vi "Day11-1.vi"() -> ()   [LabVIEW 2021]
panel:
  out "Flashes":i32
  out "Array":i32[][](array[numeric])
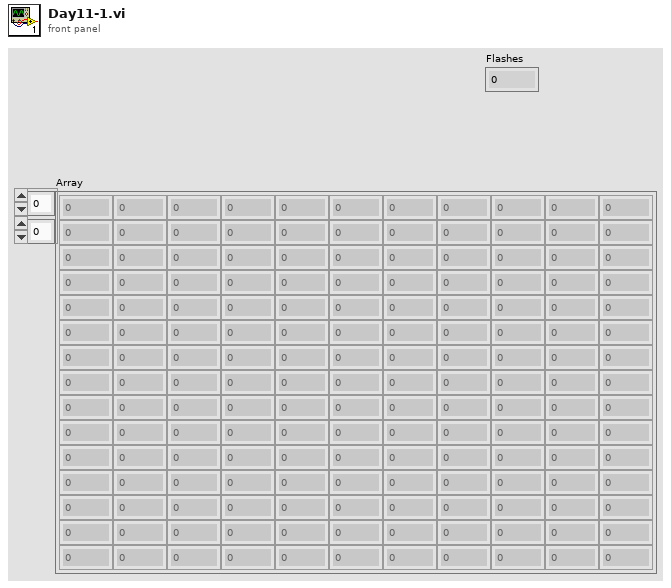
[diagram p1: front panel]
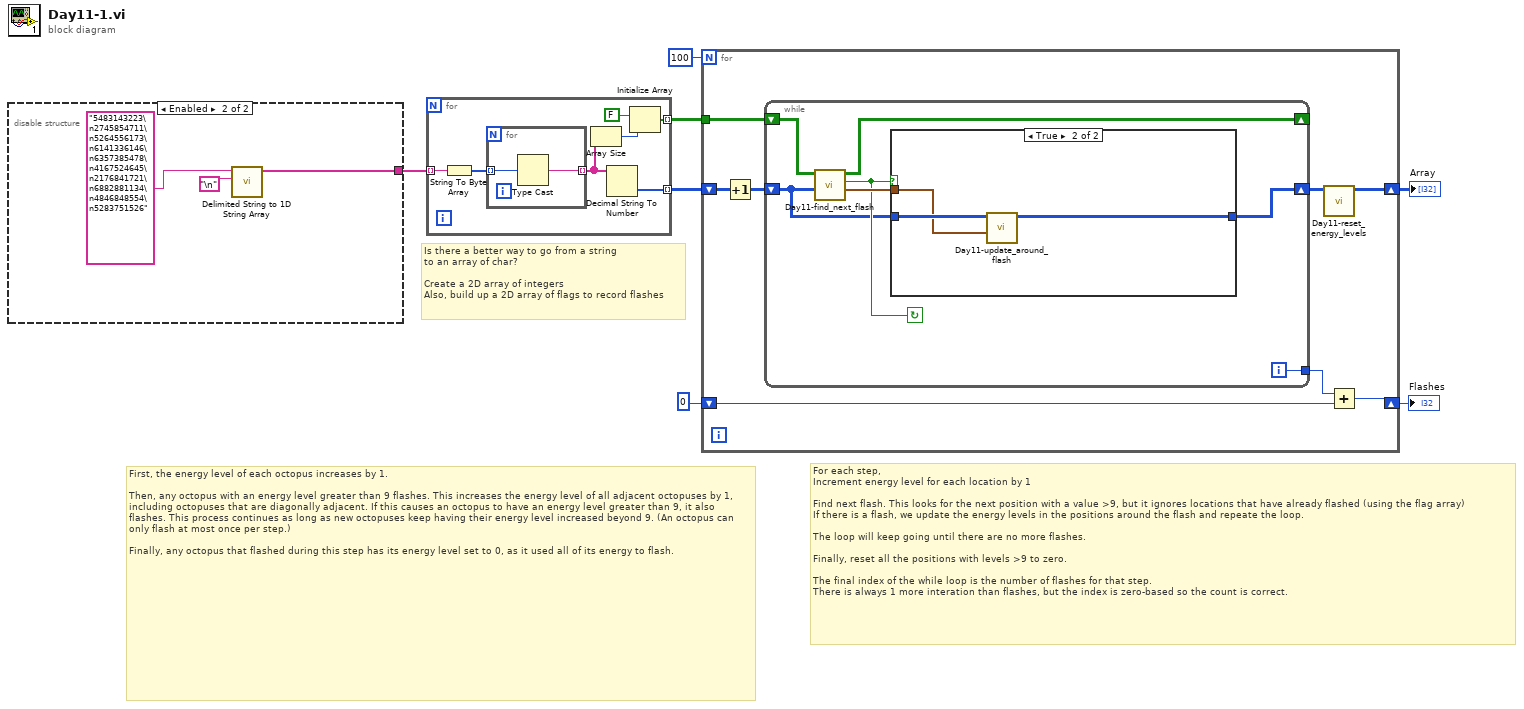
[diagram p0: block diagram]
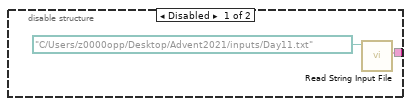
[diagram p3: hidden frame]
diagram:
  # "For each step,\nIncrement energy level for each location by 1\n\nFind next flash. This looks for the next position with a value >9, but it ignores locations that have already flashed (using the flag array)\nIf there is a flash, we update the energy levels in the positions around the flash and repeate the loop.\n\nThe loop will keep going until there are no more flashes.\n\nFinally, reset all the positions with levels >9 to zero. \n\nThe final index of the while loop is the number of flashes for that step. \nThere is always 1 more interation than flashes, but the index is zero-based so the count is correct."
  # "Is there a better way to go from a string\nto an array of char?\n\nCreate a 2D array of integers\nAlso, build up a 2D array of flags to record flashes"
  # "First, the energy level of each octopus increases by 1.\n\nThen, any octopus with an energy level greater than 9 flashes. This increases the energy level of all adjacent octopuses by 1, including octopuses that are diagonally adjacent. If this causes an octopus to have an energy level greater than 9, it also flashes. This process continues as long as new octopuses keep having their energy level increased beyond 9. (An octopus can only flash at most once per step.)\n\nFinally, any octopus that flashed during this step has its energy level set to 0, as it used all of its energy to flash."
  n1 = disable-structure shown="Enabled" {
    disable-tunnel: [w8 w10] -> w7
    frame Disabled {
      n2 = call "Read String Input File.vi"("file path (dialog if empty)"=path "C:/Users/z0000opp/Desktop/Advent2021/inputs/Day11.txt") -> ("input values"=w8:string[])  [unwired: 10 in]
    }
    frame Enabled {
      n3 = call <vilib>:"Delimited String to 1D String Array.vi"("delimiter"="\n", "delimited string"="5483143223\n2745854711\n5264556173\n6141336146\n6357385478\n4167524645\n2176841721\n6882881134\n4846848554\n5283751526") -> ("string array"=w10:string[])  [unwired: 9 in]
    }
  }
  n4 = for {
    tunnel: w7 -> [w19] mode=indexing
    tunnel: [w17] -> w5 mode=indexing
    tunnel: [w13] -> w3 mode=indexing
    n5 = String To Byte Array(string=w19) -> (unsigned byte array=w18:u8[])
    n6 = for {
      tunnel: w18 -> [w21] mode=indexing
      tunnel: [w20] -> w15 mode=indexing
      n7 = Type Cast(x=w21) -> (*(type *) &x=w20:string)  [unwired: 1 in]
    }
    n8 = Array Size(array=w15) -> (size(s)=w14:i32)
    n9 = Decimal String To Number(string=w15) -> (number=w17:i32[])  [unwired: 2 in, 1 out]
    n10 = Initialize Array(FALSE, w14) -> (w13:bool[])
  }
  n11 = for {
    N: 100 -> [_]
    shift-right: [w25] -> w4
    shift-left: w5 -> [w29]
    tunnel: w3 -> [w27]
    shift-right: [w22] -> w1
    shift-left: 0 -> [w23]
    n12 = Increment(x=w29) -> (x+1=w28:i32[][])
    n13 = while {
      shift-right: [w31] -> w26
      shift-left: w28 -> [w32]
      shift-right: [w35] -> _
      shift-left: w27 -> [w36]
      tunnel: [w30] -> w24
      i -> [w30]
      stop <- w33 continue-if-true
      n14 = call "Day11-find_next_flash.vi"("Energy Levels"=w32, "Flashed"=w36) -> ("Flash Location"=w34:cluster{i32, i32}, "New Flash?"=w33:bool, "Flashed out"=w35:bool[][])  [unwired: 7 in]
      n15 = case shown="True" w33 {
        tunnel: w34 -> [_ w39]
        tunnel: w32 -> [w37 w40]
        tunnel: [w37 w38] -> w31
        frame False {
        }
        frame True {
          n16 = call "Day11-update_around_flash.vi"("Flash Location"=w39, "Energy Levels"=w40) -> ("Energy Levels out"=w38:i32[][])  [unwired: 9 in]
        }
      }
    }
    n17 = call "Day11-reset_energy_levels.vi"("Energy Levels"=w26) -> ("Energy Levels out"=w25:i32[][])  [unwired: 10 in]
    n18 = Add(x=w24, y=w23) -> (x+y=w22:i32)
  }
  "Array" <- w4
  "Flashes" <- w1
